vi "Cannon Modifications.vi"(1 "Cannon Info":T1, 2 "InTake Max":bool) -> (0 "Cannon Info":T1)   [LabVIEW 2013]
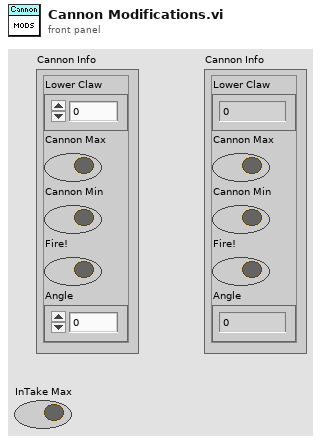
[diagram p1: front panel]
types:
  T1 = cluster{"Lower Claw":dbl, "Cannon Max":bool, "Cannon Min":bool, "Fire!":bool, "Angle":dbl}
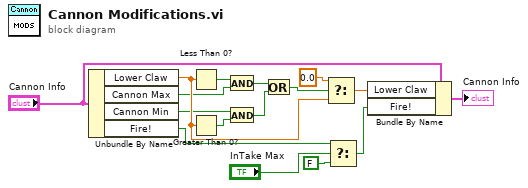
[diagram p0: block diagram]
diagram:
  n1 = Unbundle By Name("Cannon Info") -> ("Lower Claw"=w9:dbl, "Cannon Max"=w2:bool, "Cannon Min"=w3:bool, "Fire!"=w8:bool)
  n2 = Less Than 0?(x=w9) -> (x < 0?=w11:bool)
  n3 = Greater Than 0?(x=w9) -> (x > 0?=w14:bool)
  n4 = And(x=w11, y=w2) -> (x .and. y?=w13:bool)
  n5 = And(x=w3, y=w14) -> (x .and. y?=w12:bool)
  n6 = Or(x=w13, y=w12) -> (x .or. y?=w10:bool)
  n7 = Select(t=0.0, s=w10, f=w9) -> (s? t:f=w7:dbl)
  n8 = Select(t=w8, s="InTake Max", f=FALSE) -> (s? t:f=w6:bool)
  n9 = Bundle By Name(cluster="Cannon Info", "Lower Claw"=w7, "Fire!"=w6) -> (→"Cannon Info":T1)
